vi "UI Initialize.vi"(8 "error in (no error)":errorcluster, 11 "UI ActorTop in":refnum<class "UI_Tree.lvclass">) -> (0 "error out":errorcluster, 3 "UI ActorTop out":refnum<class "UI_Tree.lvclass">)   [LabVIEW 2021, in "UI_Tree.lvlib" / "UI_Tree.lvclass"]
doc: "UI: Initialize\n2015-03-18 16:27:22\n蒋松\njiangsong@outlook.com"
uses:
  UI_Tree.lvclass
  C:/Program Files (x86)/National Instruments/LabVIEW 2021/user.lib/John_Lib/AbstractActorTemplate/AbstractActorTemplate/UIActorTop.lvclass
  <vilib>/ActorFramework/Message Enqueuer/Message Enqueuer.lvclass
  <userlib>/John_Lib/Interfaces/InsertLeftSubPanel Messages/Insert Left SubPanel Msg/Insert Left SubPanel Msg.lvclass/Insert Left SubPanel Msg.ctl
  <vilib>/ActorFramework/Message Enqueuer/Message Enqueuer.lvclass/Message Enqueuer.ctl
  <vilib>/ActorFramework/Message Enqueuer/Enqueue.vi
  <userlib>/John_Lib/Interfaces/InsertLeftSubPanel Messages/Insert Left SubPanel Msg/Insert Left SubPanel Msg.lvclass
  C:/Program Files (x86)/National Instruments/LabVIEW 2021/vi.lib/ActorFramework/Message/Message.lvclass
  <vilib>/ActorFramework/Message Priority Queue/Priority Enqueue.vi
  <userlib>/John_Lib/AbstractActorTemplate/AbstractActorTemplate/UIActorTop.lvclass
  UI_Tree.lvclass/UI_Tree.ctl
  C:/Program Files (x86)/National Instruments/LabVIEW 2021/vi.lib/ActorFramework/Actor/Actor.lvclass
  C:/Program Files (x86)/National Instruments/LabVIEW 2021/project/Create Actor from Template/_UI_Tree/UI_Tree.lvclass
panel:
  out "Enqueuer":T1(c390)
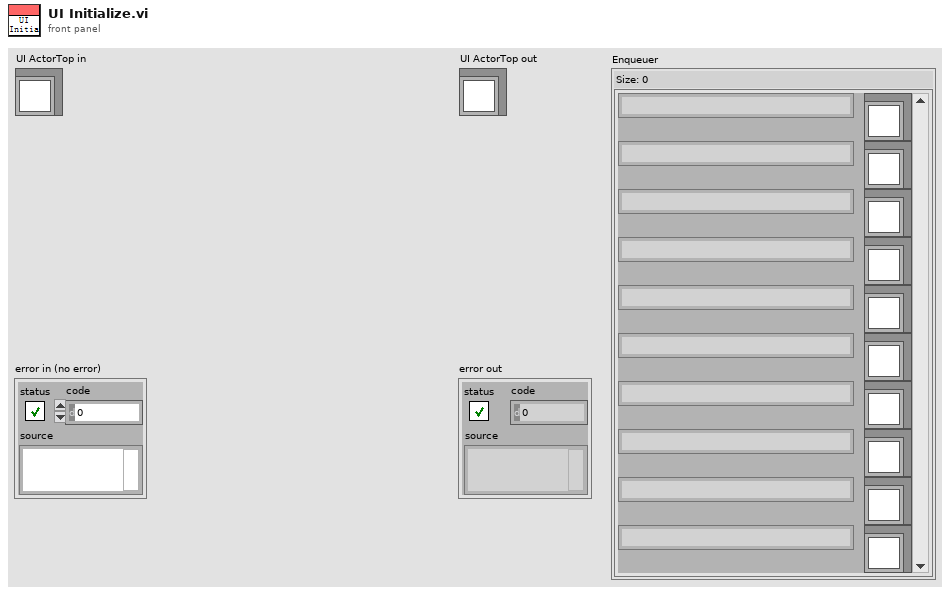
[diagram p1: front panel]
types:
  T1 = map{string, refnum<class "Message Enqueuer.lvclass">}
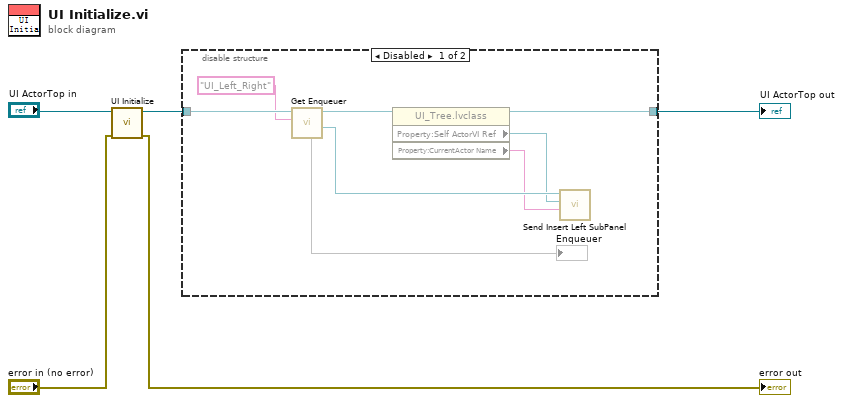
[diagram p0: block diagram]
diagram:
  n1 = call-parent "UI Initialize.vi"("error in (no error)"="error in (no error)", "UI ActorTop in"="UI ActorTop in") -> ("error out"=→"error out":errorcluster, "UI ActorTop out"=w2:refnum<class "UI_Tree.lvclass">)  [unwired: 8 in]
  n2 = disable-structure shown="Disabled" {
    disable-tunnel: w2 -> [w13 w14]
    disable-tunnel: [w9 w14] -> w1
    frame Disabled {
      n3 = call <userlib>:"Get Enqueuer.vi"("ActorQName"="UI_Left_Right", "UIActorTop in"=w13) -> ("Nested Actor's Enqueuer"=w10:refnum<class "Message Enqueuer.lvclass">, "UIActorTop in"=w12:refnum<class "UI_Tree.lvclass">, "Enqueuer"=→"Enqueuer":T1)  [unwired: 3 in, 4 out]
      n4 = property class="UI_Tree.lvclass"(reference=w12) -> (reference out=w9:refnum<class "UI_Tree.lvclass">, "Property:Self ActorVI Ref"=w8:refnum<vi>, "Property:CurrentActor Name"=w7:string)  [unwired: 1 in, 1 out]
      n5 = call <userlib>:"Send Insert Left SubPanel.vi"("ActorQName"=w7, "ActorVI Ref"=w8, "Message Enqueuer"=w10) -> ()  [unwired: 7 in, 2 out]
    }
    frame Enabled {
    }
  }
  "UI ActorTop out" <- w1
